vi "uti_GetNestedQ(NestedName).vi"(8 "error in (no error)":errorcluster, 10 "Nested Name":string, 11 "UI_Actor in":refnum<class "UI_Actor.lvclass">) -> (0 "error out":errorcluster, 2 "Nested Q":refnum<class "Message Enqueuer.lvclass">, 3 "UI_Actor out":refnum<class "UI_Actor.lvclass">)   [LabVIEW 2020, in "UI_Actor.lvlib" / "UI_Actor.lvclass"]
uses:
  UI_Actor.lvclass
  support/Actor Framework.lvlibp/1abvi3w/vi.lib/ActorFramework/Message Enqueuer/Message Enqueuer.lvclass
  UI_Actor.lvclass/UI_Actor.ctl
  ctl_ErrorSelector.ctl
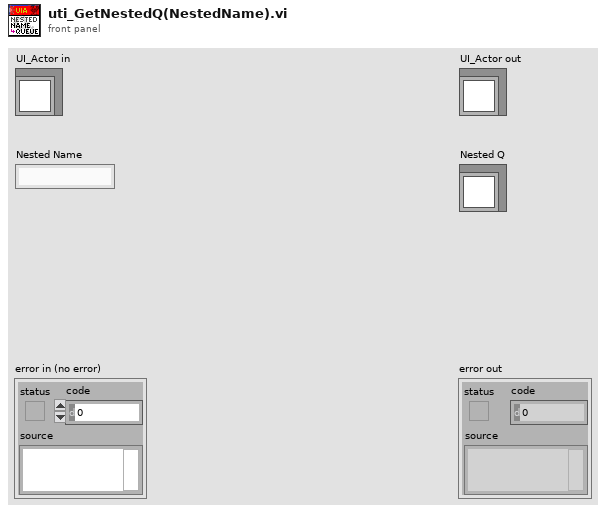
[diagram p1: front panel]
types:
  T1 = typedef "ctl_ErrorSelector.ctl" = enum16{"Unknown nested UIA", "Unsupported type"}
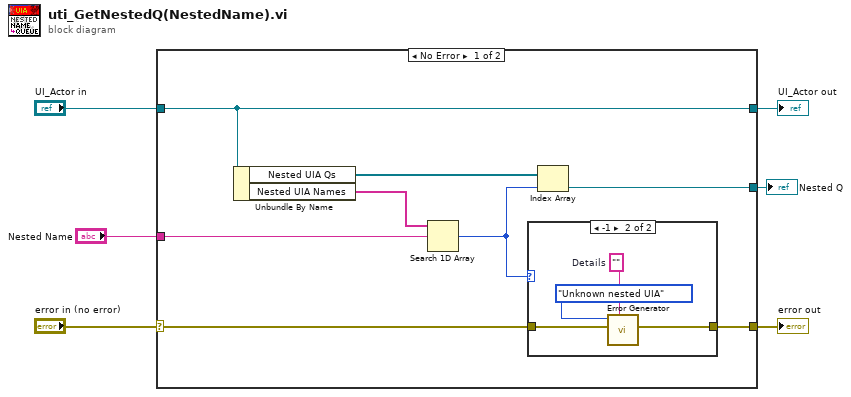
[diagram p0: block diagram]
diagram:
  n1 = case shown="No Error" "error in (no error)" {
    selector: "error in (no error)" -> [w8 w21]
    tunnel: [w7 w21] -> w5
    tunnel: [w14 w20] -> w3
    tunnel: "UI_Actor in" -> [w14 w20]
    tunnel: "Nested Name" -> [w11 _]
    tunnel: [w10 _] -> w1
    frame No Error {
      n2 = Unbundle By Name(w14) -> ("Nested UIA Qs"=w13:refnum<class "Message Enqueuer.lvclass">[], "Nested UIA Names"=w12:string[])
      n3 = Search 1D Array(1D array=w12, element=w11) -> (index of element=w9:i32)  [unwired: 1 in]
      n4 = case shown="-1" w9 {
        tunnel: w8 -> [w15 w18]
        tunnel: [w15 w17] -> w7
        frame Default {
        }
        frame -1 {
          w16 = ""  # Details
          n5 = call "Error Generator.vi"("Details"=w16, "error in (no error)"=w18, "Error selector"=ctl_ErrorSelector."Unknown nested UIA") -> ("error out"=w17:errorcluster)  [unwired: 8 in]
        }
      }
      n6 = Index Array(array=w13, index=w9) -> (element=w10:refnum<class "Message Enqueuer.lvclass">)
    }
    frame Error {
    }
  }
  "error out" <- w5
  "UI_Actor out" <- w3
  "Nested Q" <- w1
